vi "Inspect HV Pads.vi"(7 "Console Log in":refnum<class "Console Log.lvclass">, 8 "error in":errorcluster, 10 "Module Data In":T1={"TBM-TBM"={"Fiducial Image"={"Image Position"=refnum, "Image Reference"=refnum, "Field of View"={"x(mm)"=0.0, "y(mm)"=0.0}}, "Fiducials"=[]}, "TBM-HDI"={"Fiducial Image"={"Image Position"=refnum, "Image Reference"=refnum, "Field of View"={"x(mm)"=0.0, "y(mm)"=0.0}}, "Fiducials"=[]}, "Address Pads"={"Fiducial Image"={"Image Position"=refnum, "Image Reference"=refnum, "Field of View"={"x(mm)"=0.0, "y(mm)"=0.0}}, "Fiducials"=[]}, "HDI Bond Pad References"=[], "BBM Bond Pad References"=[], "HV-HDI"={"Fiducial Image"={"Image Position"=refnum, "Image Reference"=refnum, "Field of View"={"x(mm)"=0.0, "y(mm)"=0.0}}, "Selected Fiducial"={"Fiducial Image Coordinate"=refnum, "Fiducial Source"=enum."Pattern Recognition"}, "fiducial name"=""}, "HV-BBM"={"Fiducial Image"={"Image Position"=refnum, "Image Reference"=refnum, "Field of View"={"x(mm)"=0.0, "y(mm)"=0.0}}, "Selected Fiducial"={"Fiducial Image Coordinate"=refnum, "Fiducial Source"=enum."Pattern Recognition"}, "fiducial name"=""}, "Chuck"=0, "Slot"=0, "Potting Selection"={"HDI Bond Pads"=[TRUE, TRUE, TRUE, TRUE, TRUE, TRUE, TRUE, TRUE, TRUE, TRUE, TRUE, TRUE, TRUE, TRUE, TRUE, TRUE], "BBM Bond Pads"=[TRUE, TRUE, TRUE, TRUE, TRUE, TRUE, TRUE, TRUE, TRUE, TRUE, TRUE, TRUE, TRUE, TRUE, TRUE, TRUE], "TBM Inner"={"Top"=TRUE, "Left"=TRUE, "Bottom"=TRUE, "Right"=TRUE}, "TBM Outer"={"Top"=TRUE, "Left"=TRUE, "Bottom"=TRUE, "Right"=TRUE}, "Address Pads"={"Top"=TRUE, "Bottom"=TRUE}, "High Voltage"={"HDI"=TRUE, "Sensor"=TRUE}}}, 11 "Potting Procedure in":refnum<class "Potting Procedure.lvclass">) -> (0 "error out":errorcluster, 2 "Module Data Out":T1={"TBM-TBM"={"Fiducial Image"={"Image Position"=refnum, "Image Reference"=refnum, "Field of View"={"x(mm)"=0.0, "y(mm)"=0.0}}, "Fiducials"=[]}, "TBM-HDI"={"Fiducial Image"={"Image Position"=refnum, "Image Reference"=refnum, "Field of View"={"x(mm)"=0.0, "y(mm)"=0.0}}, "Fiducials"=[]}, "Address Pads"={"Fiducial Image"={"Image Position"=refnum, "Image Reference"=refnum, "Field of View"={"x(mm)"=0.0, "y(mm)"=0.0}}, "Fiducials"=[]}, "HDI Bond Pad References"=[], "BBM Bond Pad References"=[], "HV-HDI"={"Fiducial Image"={"Image Position"=refnum, "Image Reference"=refnum, "Field of View"={"x(mm)"=0.0, "y(mm)"=0.0}}, "Selected Fiducial"={"Fiducial Image Coordinate"=refnum, "Fiducial Source"=enum."Pattern Recognition"}, "fiducial name"=""}, "HV-BBM"={"Fiducial Image"={"Image Position"=refnum, "Image Reference"=refnum, "Field of View"={"x(mm)"=0.0, "y(mm)"=0.0}}, "Selected Fiducial"={"Fiducial Image Coordinate"=refnum, "Fiducial Source"=enum."Pattern Recognition"}, "fiducial name"=""}, "Chuck"=0, "Slot"=0, "Potting Selection"={"HDI Bond Pads"=[TRUE, TRUE, TRUE, TRUE, TRUE, TRUE, TRUE, TRUE, TRUE, TRUE, TRUE, TRUE, TRUE, TRUE, TRUE, TRUE], "BBM Bond Pads"=[TRUE, TRUE, TRUE, TRUE, TRUE, TRUE, TRUE, TRUE, TRUE, TRUE, TRUE, TRUE, TRUE, TRUE, TRUE, TRUE], "TBM Inner"={"Top"=TRUE, "Left"=TRUE, "Bottom"=TRUE, "Right"=TRUE}, "TBM Outer"={"Top"=TRUE, "Left"=TRUE, "Bottom"=TRUE, "Right"=TRUE}, "Address Pads"={"Top"=TRUE, "Bottom"=TRUE}, "High Voltage"={"HDI"=TRUE, "Sensor"=TRUE}}}, 3 "Potting Procedure out":refnum<class "Potting Procedure.lvclass">, 5 "Console Log out":refnum<class "Console Log.lvclass">)   [LabVIEW 2011, in "Potting Procedure.lvclass"]
uses:
  Potting Procedure.lvclass
  UI Classes/Console Log/Console Log.lvclass
  Type Definitions/Inspect Modules - Module.ctl
  Shared Components/Vec3d Class/Vec3d Class.lvclass
  Shared Components/Utils/Type Definitions/Multi-Fiducial Image.ctl
  Shared Components/Utils/Type Definitions/Physical Image.ctl
  <vilib>/vision/Image Controls.llb/IMAQ Image.ctl
  Shared Components/Utils/Type Definitions/Fiducial with Source.ctl
  Shared Components/Utils/Type Definitions/Fiducial Image.ctl
  Shared Components/Config Manager Class/Type Definitions/Part Type.ctl
  Shared Components/Gantry Class/Gantry Class.lvclass
  Shared Components/WorkTable Class/WorkTable Class.lvclass
  Shared Components/Config Manager Class/Type Definitions/Camera Enum.ctl
  Shared Components/Config Manager Class/Config Manager Class.lvclass
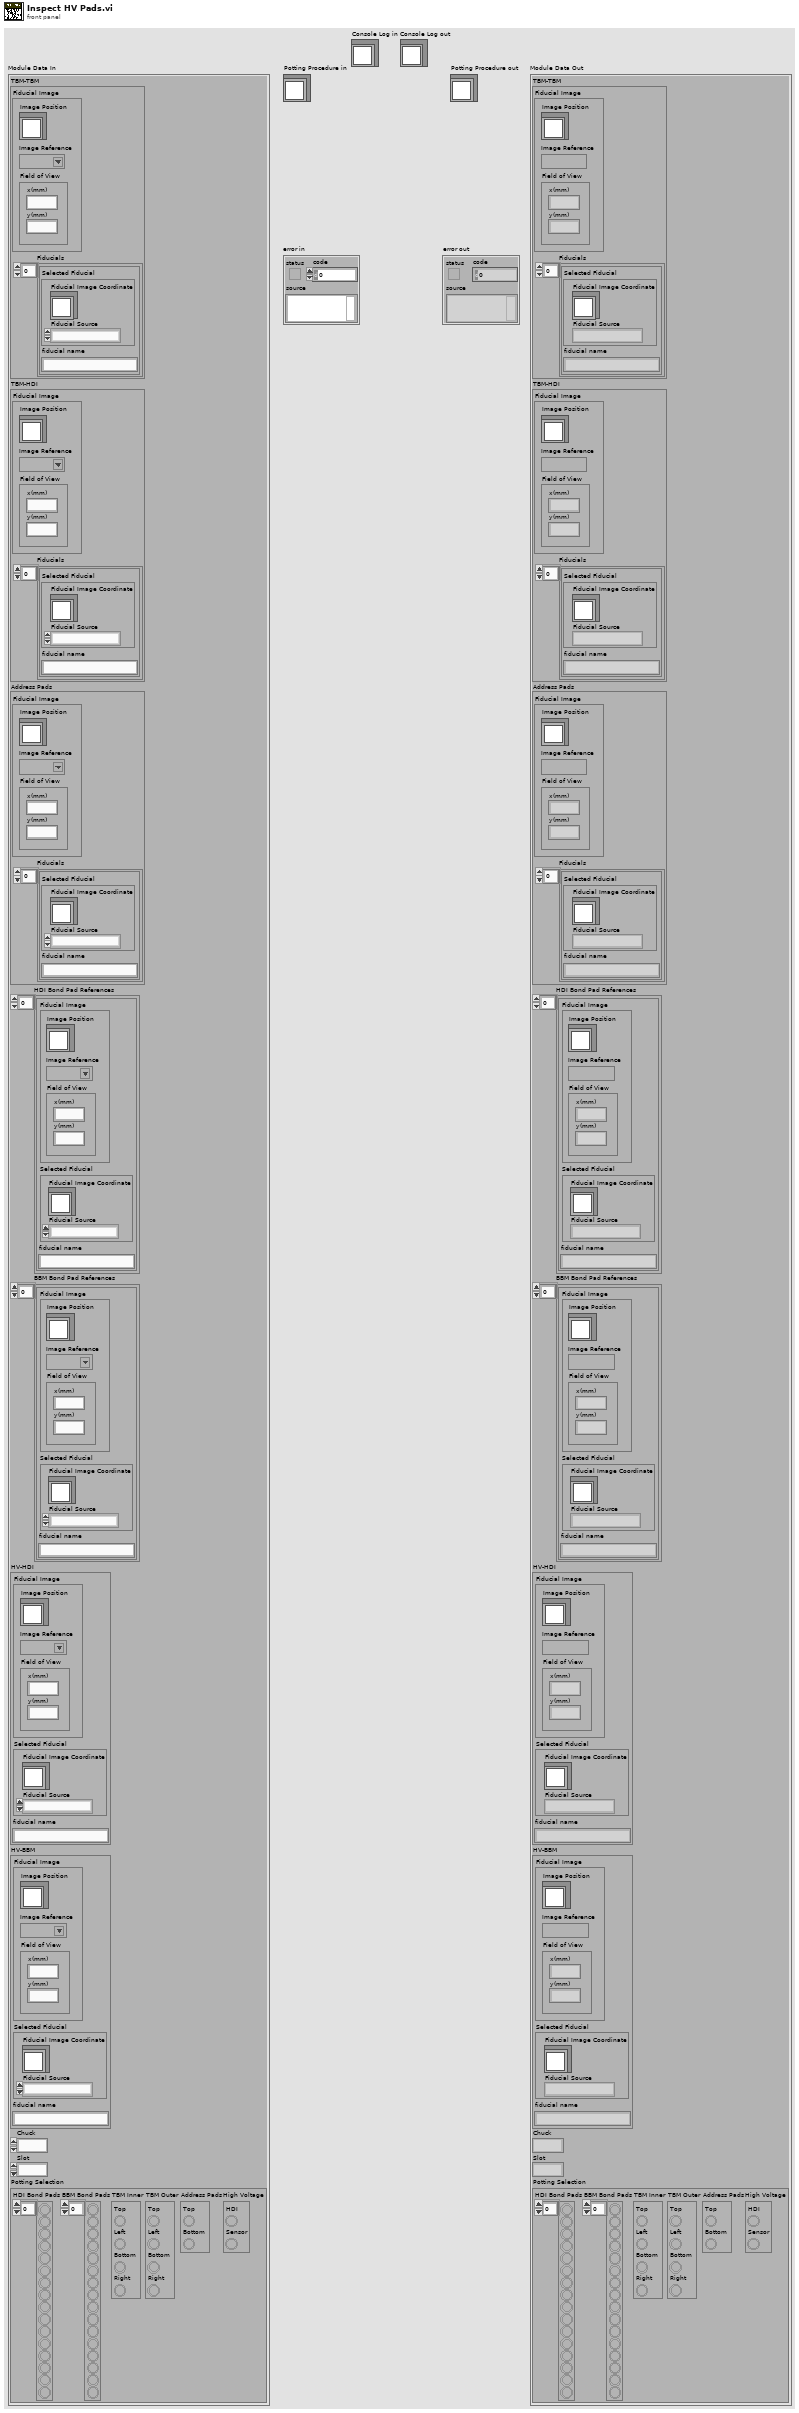
[diagram p1: front panel]
types:
  T1 = typedef "Inspect Modules - Module.ctl" = cluster{"TBM-TBM":T2, "TBM-HDI":T2, "Address Pads":T2, "HDI Bond Pad References":T6[], "BBM Bond Pad References":T6[], "HV-HDI":T6, "HV-BBM":T6, "Chuck":i32, "Slot":i32, "Potting Selection":cluster{"HDI Bond Pads":bool[], "BBM Bond Pads":bool[], "TBM Inner":cluster{"Top":bool, "Left":bool, "Bottom":bool, "Right":bool}, "TBM Outer":cluster{"Top":bool, "Left":bool, "Bottom":bool, "Right":bool}, "Address Pads":cluster{"Top":bool, "Bottom":bool}, "High Voltage":cluster{"HDI":bool, "Sensor":bool}}}
  T2 = typedef "Multi-Fiducial Image.ctl" = cluster{"Fiducial Image":T3, "Fiducials":cluster{"Selected Fiducial":T5, "fiducial name":string}[]}
  T3 = typedef "Physical Image.ctl" = cluster{"Image Position":refnum<class "Vec3d Class.lvclass">, "Image Reference":T4, "Field of View":cluster{"x(mm)":dbl, "y(mm)":dbl}}
  T4 = typedef "IMAQ Image.ctl" = refnum<image>
  T5 = typedef "Fiducial with Source.ctl" = cluster{"Fiducial Image Coordinate":refnum<class "Vec3d Class.lvclass">, "Fiducial Source":enum16{"Pattern Recognition", "User", "Error", "Default"}}
  T6 = typedef "Fiducial Image.ctl" = cluster{"Fiducial Image":T3, "Selected Fiducial":T5, "fiducial name":string}
  T7 = typedef "Part Type.ctl" = enum16{"BBM", "HDI", "GLUERESERVOIR", "STAMP", "WEIGHT"}
  T8 = typedef "Camera Enum.ctl" = enum16{"GANTRY HEAD", "NEEDLE CALIBRATION X", "NEEDLE CALIBRATION Y"}
  T9 = enum16{"Pattern Recognition", "User", "Error", "Default"}
  T10 = typedef "Worktable_Module Slot.ctl" = cluster{"Slot State":enum16{"Empty", "Unglued", "Stamped", "PartOnTop", "Weighted", "Unpotted", "Potted"}, "BBM Type":enum16{"None", "BBM", "GlassSlide"}, "HDI Type":enum16{"None", "HDI", "Polyimide"}, "Vacuum Channel":u8, "Location/Orientation BBM":T11, "Location/Orientation HDI":T11, "S/N":string}
  T11 = typedef "Position_Orientation.ctl" = cluster{"Center":refnum<class "Vec3d Class.lvclass">, "Orientation":refnum<class "Orient3d Class.lvclass">}
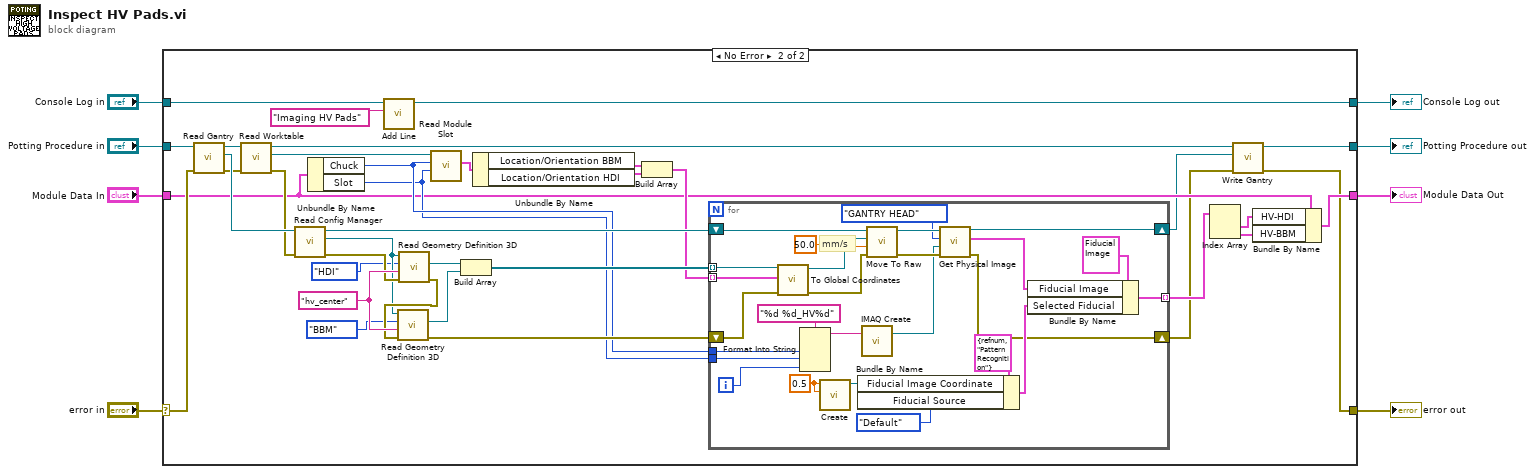
[diagram p0: block diagram]
diagram:
  n1 = case shown="No Error" "error in" {
    selector: "error in" -> [w11 w35]
    tunnel: [w11 w19] -> w7
    tunnel: [w12 w22] -> w5
    tunnel: "Potting Procedure in" -> [w12 w49]
    tunnel: [w10 w27] -> w1
    tunnel: "Module Data In" -> [w10 w28]
    tunnel: "Console Log in" -> [w9 w18]
    tunnel: [w9 w17] -> w3
    frame Error {
    }
    frame No Error {
      w46 = "hv_center" ("Feature")
      n2 = call-dynamic "Read Gantry.vi"("error in (no error)"=w35, "Potting Procedure in"=w49) -> ("error out"=w34:errorcluster, "Gantry"=w47:refnum<class "Gantry Class.lvclass">, "Potting Procedure out"=w48:refnum<class "Potting Procedure.lvclass">)  [unwired: 7 in]
      n3 = call-dynamic "Read Worktable.vi"("error in"=w34, "Potting Procedure in"=w48) -> ("error out"=w33:errorcluster, "WorkTable out"=w44:refnum<class "WorkTable Class.lvclass">, "Potting Procedure out"=w23:refnum<class "Potting Procedure.lvclass">)  [unwired: 7 in]
      n4 = call-dynamic "Read Config Manager.vi"("error in"=w33, "Gantry in"=w47) -> ("error out"=w31:errorcluster, "Config Manager"=w15:refnum<class "Config Manager Class.lvclass">, "Gantry out"=w42:refnum<class "Gantry Class.lvclass">)  [unwired: 7 in]
      n5 = Unbundle By Name(w28) -> ("Chuck"=w30:i32, "Slot"=w29:i32)
      n6 = call "Add Line.vi"("String"="Imaging HV Pads", "Console Log in"=w18) -> ("Console Log out"=w17:refnum<class "Console Log.lvclass">)  [unwired: 8 in, 1 out]
      n7 = call "Read Geometry Definition 3D.vi"("error in"=w31, "Feature"=w46, "Part Type"=Part_Type."HDI", "Config Manager in"=w15) -> ("error out"=w45:errorcluster, "Feature Coordinates"=w41:refnum<class "Vec3d Class.lvclass">)  [unwired: 5 in, 1 out]
      n8 = call "Read Geometry Definition 3D.vi"("error in"=w45, "Feature"=w46, "Part Type"=Part_Type."BBM", "Config Manager in"=w15) -> ("error out"=w32:errorcluster, "Feature Coordinates"=w40:refnum<class "Vec3d Class.lvclass">)  [unwired: 5 in, 1 out]
      n9 = call-dynamic "Read Module Slot.vi"("slot"=w29, "chuck"=w30, "WorkTable in"=w44) -> ("Module Slot"=w43:T10)  [unwired: 6 in, 2 out]
      n10 = Build Array(w41, w40) -> (w39:refnum<class "Vec3d Class.lvclass">[])
      n11 = Unbundle By Name(w43) -> ("Location/Orientation BBM"=w38:T11, "Location/Orientation HDI"=w37:T11)
      n12 = Build Array(w38, w37) -> (w36:T11[])
      n13 = for {
        tunnel: w39 -> [w74] mode=indexing
        tunnel: w36 -> [w75] mode=indexing
        shift-right: [w66] -> w21
        shift-left: w42 -> [w72]
        tunnel: w30 -> [w64]
        tunnel: w29 -> [w63]
        tunnel: [w58] -> w24 mode=indexing
        shift-right: [w51] -> w20
        shift-left: w32 -> [w73]
        i -> [w62]
        w54 = 0.5 ("X")
        # "mm/s"
        n14 = call "To Global Coordinates.vi"("error in"=w73, "Center/Orientation"=w75, "Local Coordinates"=w74) -> ("error out"=w70:errorcluster, "Global Coordinates"=w71:refnum<class "Vec3d Class.lvclass">)  [unwired: 7 in]
        n15 = Format Into String(format string="%d %d_HV%d", w64, w63, w62) -> (resulting string=w61:string)  [unwired: 2 in, 1 out]
        n16 = call "Create.vi"("Y"=w54, "X"=w54) -> ("Vec3d Class out"=w53:refnum<class "Vec3d Class.lvclass">)  [unwired: 8 in, 1 out]
        n17 = Bundle By Name(cluster=T5 {"Fiducial Image Coordinate"=refnum, "Fiducial Source"=enum."Pattern Recognition"} ("Selected Fiducial"), "Fiducial Image Coordinate"=w53, "Fiducial Source"=T9."Default") -> (w55:T5)
        n18 = call "IMAQ Create"("Image Name"=w61) -> ("New Image"=w60:T4)  [unwired: 4 in, 1 out]
        n19 = call-dynamic "Move To Raw.vi"("error in"=w70, "Speed"=50.0, "Destination"=w71, "Gantry in"=w72) -> ("error out"=w67:errorcluster, "Gantry out"=w68:refnum<class "Gantry Class.lvclass">)  [unwired: 6 in]
        n20 = call-dynamic "Get Physical Image.vi"("error in"=w67, "Image In"=w60, "Camera Name"=Camera_Enum."GANTRY HEAD", "Gantry in"=w68) -> ("error out"=w51:errorcluster, "Physical Image"=w57:T3, "Gantry out"=w66:refnum<class "Gantry Class.lvclass">)  [unwired: 5 in]
        n21 = Bundle By Name(cluster=T6 {"Fiducial Image"={"Image Position"=refnum, "Image Reference"=refnum, "Field of View"={"x(mm)"=0.0, "y(mm)"=0.0}}, "Selected Fiducial"={"Fiducial Image Coordinate"=refnum, "Fiducial Source"=enum."Pattern Recognition"}, "fiducial name"=""} ("HV-TBM"), "Fiducial Image"=w57, "Selected Fiducial"=w55) -> (w58:T6)
      }
      n22 = Index Array(array=w24) -> (element #1=w26:T6, element #2=w25:T6)  [unwired: 2 in]
      n23 = call-dynamic "Write Gantry.vi"("error in (no error)"=w20, "Gantry"=w21, "Potting Procedure in"=w23) -> ("error out"=w19:errorcluster, "Potting Procedure out"=w22:refnum<class "Potting Procedure.lvclass">)  [unwired: 7 in]
      n24 = Bundle By Name(cluster=w28, "HV-HDI"=w26, "HV-BBM"=w25) -> (w27:T1)
    }
  }
  "error out" <- w7
  "Potting Procedure out" <- w5
  "Console Log out" <- w3
  "Module Data Out" <- w1
